vi "Read Timeout Serial.vi"(8 "error in":errorcluster, 11 "VISA Interface in":refnum<class "VISA Interface.lvclass">) -> (0 "error out":errorcluster, 2 "Timeout Serial":u32=10000, 3 "VISA Interface out":refnum<class "VISA Interface.lvclass">)   [LabVIEW 2020, in "Plugin Instrument Driver.lvlib" / "VISA Interface.lvclass"]
doc: "Read Timeout Serial"
uses:
  VISA Interface.lvclass
  VISA Interface.lvclass/VISA Interface.ctl
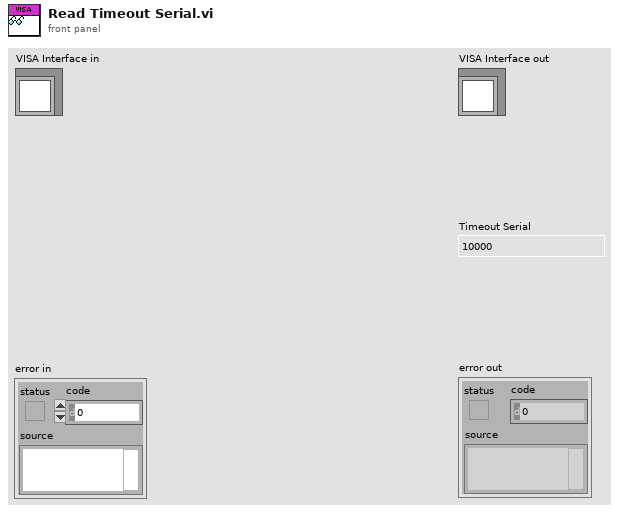
[diagram p1: front panel]
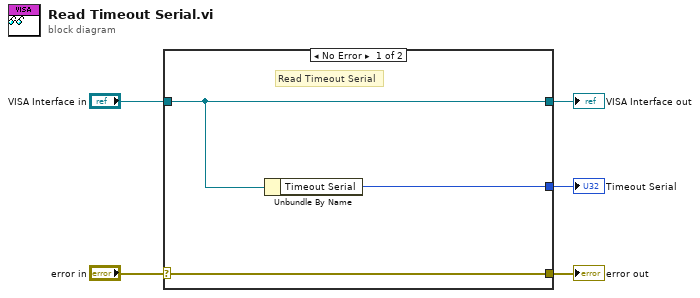
[diagram p0: block diagram]
diagram:
  n1 = case shown="No Error" "error in" {
    selector: "error in" -> [w8 w9]
    tunnel: [w8 w9] -> w4
    tunnel: [w7 w10] -> w2
    tunnel: "VISA Interface in" -> [w7 w10]
    tunnel: [w6 _] -> w1
    frame No Error {
      # "Read Timeout Serial"
      n2 = Unbundle By Name(w7) -> ("Timeout Serial"=w6:u32)
    }
    frame Error {
    }
  }
  "error out" <- w4
  "VISA Interface out" <- w2
  "Timeout Serial" <- w1
